vi "Read configuration.vi"(8 "error in":errorcluster, 11 "Daqmx Module editor node in":refnum<class "Daqmx Module editor node.lvclass">) -> (0 "error out":errorcluster, 2 "configuration":refnum<class "NISE_CEF_serializable configuration.lvclass">, 3 "Daqmx Module editor node out":refnum<class "Daqmx Module editor node.lvclass">)   [LabVIEW 2014, in "Daqmx Module editor node.lvclass"]
uses:
  Daqmx Module editor node.lvclass
  <vilib>/NI/Configuration Framework/serializable configuration/NISE_CEF_serializable configuration.lvclass
  Daqmx Module editor node.lvclass/Daqmx Module editor node.ctl
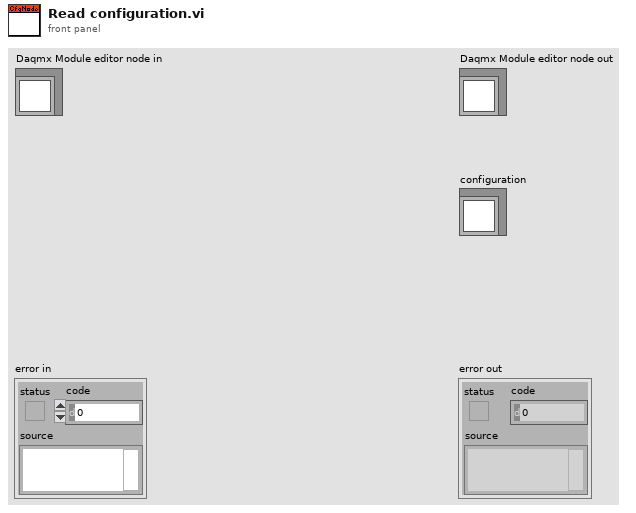
[diagram p1: front panel]
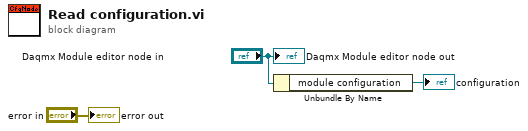
[diagram p0: block diagram]
diagram:
  n1 = Unbundle By Name("Daqmx Module editor node in") -> ("module configuration"=→"configuration":refnum<class "Daqmx Module configuration.lvclass">)
  "error out" <- "error in"
  "Daqmx Module editor node out" <- "Daqmx Module editor node in"
